vi "init manipulator.vi"(8 "error in":errorcluster, 11 "Actuator cluster in":T1={"Actuator COM"="COM14", "Actuator type"=enum."Scientifica"}) -> (0 "error out":errorcluster, 1 "angle string out":string, 2 "initialization error":bool, 3 "Actuator cluster out":T1={"Actuator COM"="COM14", "Actuator type"=enum."Scientifica"})   [LabVIEW 2015]
uses:
  pipette cleaning/pressure box/cleaning_soft/controls/scientifica_commands.ctl
  pipette cleaning/pressure box/cleaning_soft/controls/actuator_type.ctl
  pipette cleaning/pressure box/cleaning_soft/controls/actuator_cluster.ctl
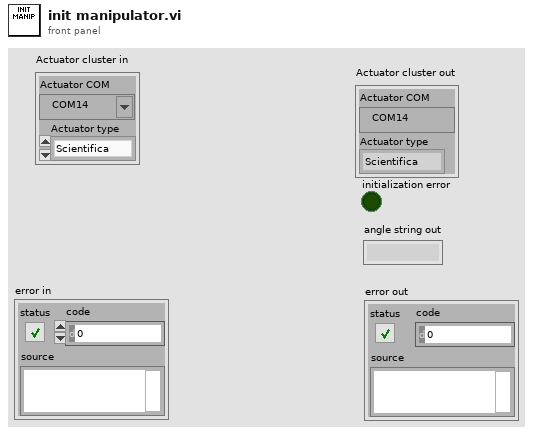
[diagram p1: front panel]
types:
  T1 = typedef "actuator_cluster.ctl" = cluster{"Actuator COM":refnum<visa-resource-name>, "Actuator type":T2}
  T2 = typedef "actuator_type.ctl" = enum16{"Scientifica", "Sutter", "Demo", "Off"}
  T3 = typedef "scientifica_commands.ctl" = enum16{"ANGLE", "INSET", "FIRST", "ZERO", "Pz", "P", "absz", "ACC", "TOP", "STOP", "rel", "relz", "abs", "IN", "vj", "APROACH", "OBJS", "OBJU", "OUT", "OBJ", "OBJL", "SET", "OBJD", "STEP", "SETSTEP", "S", "UUX", "UUY", "UUZ"}
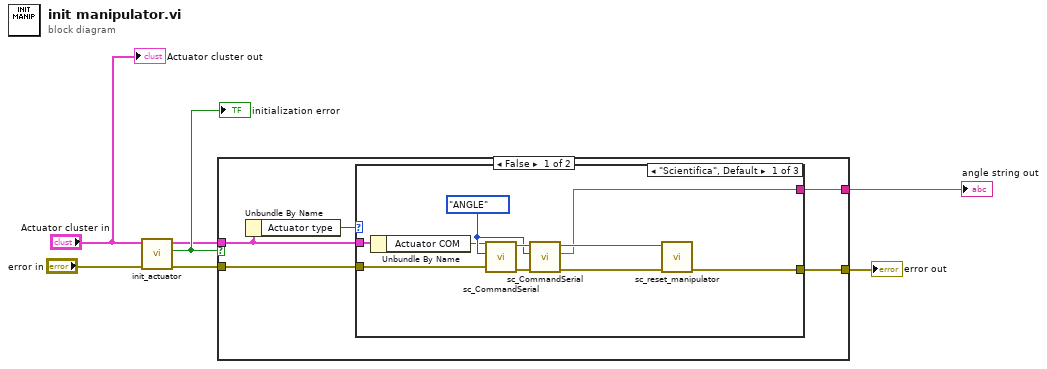
[diagram p0: block diagram]
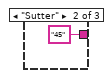
[diagram p2: hidden frame]
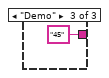
[diagram p3: hidden frame]
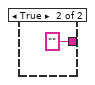
[diagram p4: hidden frame]
diagram:
  n1 = call "init_actuator.vi"("error in"="error in", "Actuator cluster in"="Actuator cluster in") -> ("error out"=w4:errorcluster, "initialization error"=w6:bool, "Actuator cluster out"=w5:T1)  [unwired: 7 in]
  "initialization error" <- w6
  n2 = case shown="False" w6 {
    tunnel: w5 -> [w11 _]
    tunnel: w4 -> [w10 _]
    tunnel: [w9 "" ("Response")] -> w3
    tunnel: [w8 _] -> w1
    frame False {
      n3 = Unbundle By Name(w11) -> ("Actuator type"=w12:T2)
      n4 = case shown="\"Scientifica\", Default" w12 {
        tunnel: w11 -> [w15 _ _]
        tunnel: w10 -> [w16 _ _]
        tunnel: [w17 "45" ("Response") "45" ("Response")] -> w9
        tunnel: [w13 _ _] -> w8
        frame "Scientifica", Default {
          w20 = scientifica_commands."ANGLE" ("Scientifica commands")
          n5 = Unbundle By Name(w15) -> ("Actuator COM"=w14:refnum<visa-resource-name>)
          n6 = call "sc_CommandSerial.vi"("error in (no error)"=w16, "Scientifica commands"=w20, "VISA handle"=w14) -> ("error out"=w21:errorcluster, "Dup. VISA handle"=w22:refnum<visa-resource-name>)  [unwired: 5 in, 2 out]
          n7 = call "sc_CommandSerial.vi"("error in (no error)"=w21, "Scientifica commands"=w20, "VISA handle"=w22) -> ("error out"=w18:errorcluster, "Response"=w17:string, "Dup. VISA handle"=w19:refnum<visa-resource-name>)  [unwired: 5 in, 1 out]
          n8 = call "sc_reset_manipulator.vi"("error in (no error)"=w18, "visa in"=w19) -> ("error out"=w13:errorcluster)  [unwired: 8 in, 1 out]
        }
        frame "Sutter" {
        }
        frame "Demo" {
        }
      }
    }
    frame True {
    }
  }
  "angle string out" <- w3
  "error out" <- w1
  "Actuator cluster out" <- "Actuator cluster in"
